vi "Configure Memory Handling.vi"(8 "error in (no error)":errorcluster, 10 "Memory Full Handling Policy (0:Stop)":u16(ring) items=["Stop", "Overwrite", "Automatic"], 11 "VISA resource name":refnum<visa-resource-name>) -> (0 "error out":errorcluster, 3 "VISA resource name out":refnum<visa-resource-name>)   [LabVIEW 2013, in "Watts Up Series.lvlib"]
doc: "Determines how new data will be recorded once the internal memory has filled up."
uses:
  <instrlib>/Watts Up Series/Watts Up Series.lvlib
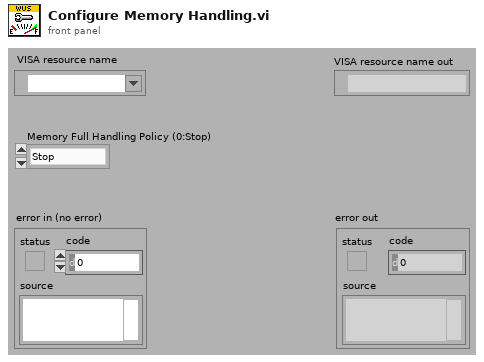
[diagram p1: front panel]
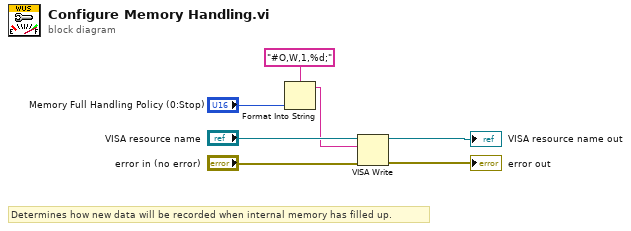
[diagram p0: block diagram]
diagram:
  # "Determines how new data will be recorded when internal memory has filled up."
  n1 = Format Into String(format string="#O,W,1,%d;", "Memory Full Handling Policy (0:Stop)") -> (resulting string=w1:string)  [unwired: 2 in, 1 out]
  n2 = VISA Write(VISA resource name="VISA resource name", write buffer=w1, error in (no error)="error in (no error)") -> (VISA resource name out=→"VISA resource name out":refnum<visa-resource-name>, error out=→"error out":errorcluster)  [unwired: 1 out]
